vi "Load Images from File.vi"(6 "Force Load":bool, 8 "Images":i32, 9 "image files":string[](array[string]), 10 "Folder Location":path, 11 "Refnum in":T1) -> (0 "error out":errorcluster, 3 "Refnum out":T1)   [LabVIEW 2023]
uses:
  <vilib>/vision/Image Controls.llb/IMAQ Image.ctl
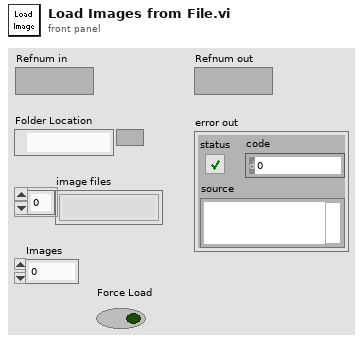
[diagram p1: front panel]
types:
  T1 = typedef "IMAQ Image.ctl" = refnum<image>
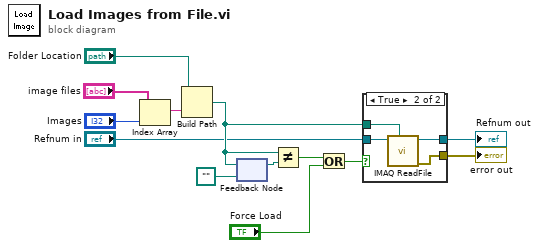
[diagram p0: block diagram]
diagram:
  n1 = Index Array(array="image files", index="Images") -> (element=w8:string)
  n2 = Build Path(base path="Folder Location", name or relative path=w8) -> (appended path=w12:path)
  n3 = feedback #1(path "" ("appended path")) -> (w10:path)
  n4 = feedback-in #1(w12) -> ()
  n5 = Not Equal?(x=w12, y=w10) -> (x != y?=w2:bool)
  n6 = Or(x=w2, y="Force Load") -> (x .or. y?=w1:bool)
  n7 = case shown="True" w1 {
    tunnel: [w14 w18] -> w4
    tunnel: [_ w17] -> w5
    tunnel: "Refnum in" -> [w14 w16]
    tunnel: w12 -> [_ w15]
    frame False {
    }
    frame True {
      n8 = call "IMAQ ReadFile"("File Path"=w15, "Image"=w16) -> ("error out"=w17:errorcluster, "Image Out"=w18:T1)  [unwired: 5 in, 3 out]
    }
  }
  "error out" <- w5
  "Refnum out" <- w4
